vi "etc_XCITE_SetLogMode.vi"(8 "error in (no error)":errorcluster {"code" format="%x"}, 11 "mode":i32) -> (0 "error out":errorcluster {"code" format="%x"})   [LabVIEW 2019, in "XCite.lvlib"]
doc: "Sends a command to execute on the slelected X-cite device."
uses:
  XCite.lvlib
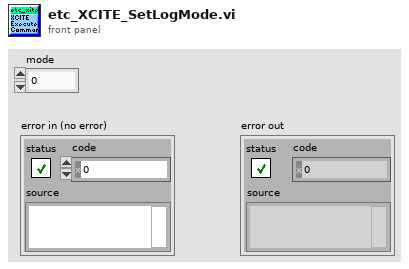
[diagram p1: front panel]
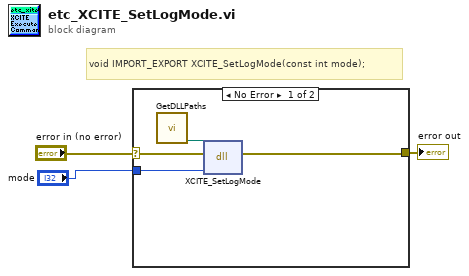
[diagram p0: block diagram]
diagram:
  # "void IMPORT_EXPORT XCITE_SetLogMode(const int mode);"
  n1 = case shown="No Error" "error in (no error)" {
    selector: "error in (no error)" -> [w7 w8]
    tunnel: [w4 w8] -> w3
    tunnel: "mode" -> [w5 _]
    frame No Error {
      n2 = call "GetDLLPaths.vi"() -> ("etc_xcite_path"=w6:path)  [unwired: 8 in, 3 out]
      n3 = dll-call lib="C:/LabVIEWDevFall2024/pco.labview/labview_sdk/runtime/bin64/etc_xcite.dll" fn="XCITE_SetLogMode"(path in=w6, error in=w7, "mode"=w5) -> (error out=w4:errorcluster)  [unwired: 3 in, 1 out]
    }
    frame Error {
    }
  }
  "error out" <- w3
